vi "Decode Key.vi"(9 "PlatMods":T1, 10 "Mods":cluster{"Num Pad":bool, "Menu Key":bool}, 11 "ScanCode":i16) -> (3 "Key":string)   [LabVIEW 2021, in "Seq Edit Quick Drop.lvlib"]
uses:
  Seq Edit Quick Drop.lvlib
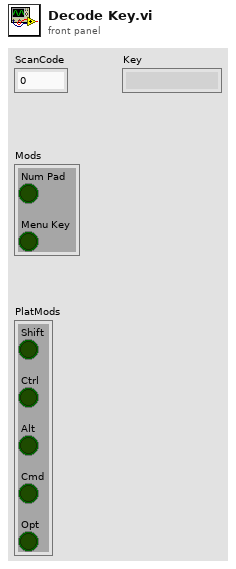
[diagram p1: front panel]
types:
  T1 = cluster{"Shift":bool, "Ctrl":bool, "Alt":bool, "Cmd":bool, "Opt":bool}
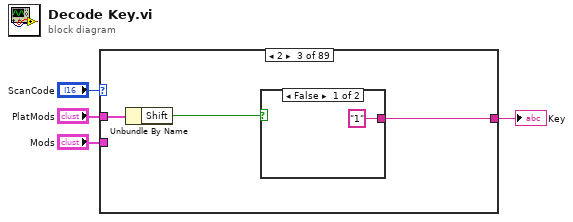
[diagram p0: block diagram]
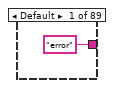
[diagram p2: hidden frame]
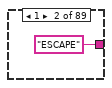
[diagram p3: hidden frame]
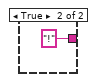
[diagram p4: hidden frame]
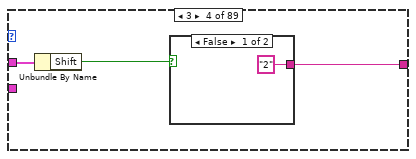
[diagram p5: hidden frame]
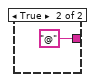
[diagram p6: hidden frame]
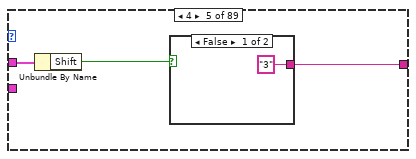
[diagram p7: hidden frame]
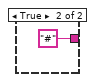
[diagram p8: hidden frame]
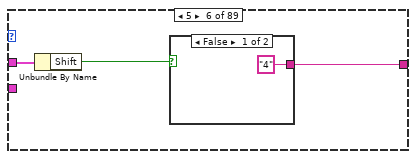
[diagram p9: hidden frame]
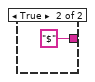
[diagram p10: hidden frame]
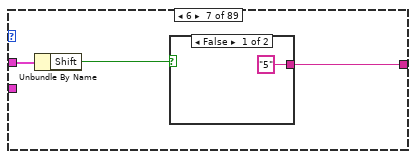
[diagram p11: hidden frame]
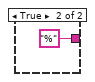
[diagram p12: hidden frame]
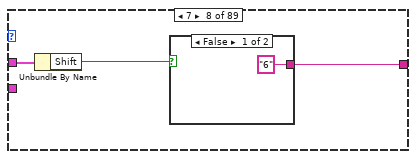
[diagram p13: hidden frame]
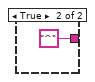
[diagram p14: hidden frame]
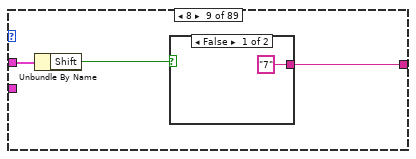
[diagram p15: hidden frame]
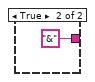
[diagram p16: hidden frame]
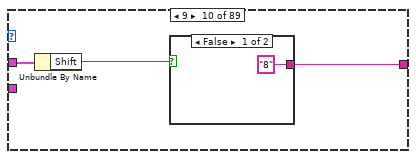
[diagram p17: hidden frame]
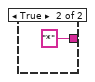
[diagram p18: hidden frame]
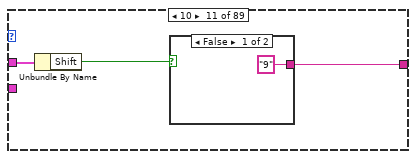
[diagram p19: hidden frame]
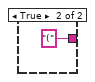
[diagram p20: hidden frame]
diagram:
  n1 = case shown="2" "ScanCode" {
    tunnel: ["error" "ESCAPE" w8 w13 w19 w24 w29 w32 w39 w44 w49 w54 w58 w62 "backspace" "tab" w70 w75 w80 w84 w89 w94 w99 w104 w109 w114 w119 w124 "Enter" "control" w132 w137 w142 w147 w152 w157 w162 w167 w172 w177 w181 w186 "LSHIFT" w193 w197 w203 w208 w212 w217 w222 w227 w232 w237 w243 "RSHIFT" w250 "RSHIFT" "SPACE" "CAPSLOCK" "F1" "F2" "F3" "F4" "F5" "F6" "F7" "F8" "F9" "F10" "numlock" "error" w269 w275 w278 "-" w284 "5" w290 "+" w296 w301 w306 w313 w318 "F11" "F12" "left win key" "right win key" "select"] -> w2
    tunnel: "Mods" -> [_ _ _ _ _ _ _ _ _ _ _ _ _ _ _ _ _ _ _ _ _ _ _ _ _ _ _ _ _ _ _ _ _ _ _ _ _ _ _ _ _ _ _ _ _ _ _ _ _ _ _ _ _ _ _ w248 _ _ _ _ _ _ _ _ _ _ _ _ _ _ _ w268 w274 w279 _ w285 _ w291 _ w297 w302 w307 w311 w316 _ _ _ _ _]
    tunnel: "PlatMods" -> [_ _ w9 w12 w17 w22 w27 w33 w37 w42 w47 w52 w57 w63 _ _ w69 w74 w79 w85 w90 w95 w100 w105 w110 w115 w120 w125 _ _ w131 w136 w141 w146 w151 w156 w161 w166 w171 w176 w182 w187 _ w192 w198 w202 w207 w213 w218 w223 w228 w233 w238 w242 _ _ _ _ _ _ _ _ _ _ _ _ _ _ _ _ _ _ _ _ _ _ _ _ _ _ _ _ _ _ _ _ _ _ _]
    frame Default {
    }
    frame 1 {
    }
    frame 2 {
      n2 = Unbundle By Name(w9) -> ("Shift"=w7:bool)
      n3 = case shown="False" w7 {
        tunnel: ["1" "!"] -> w8
        frame False {
        }
        frame True {
        }
      }
    }
    frame 3 {
      n4 = Unbundle By Name(w12) -> ("Shift"=w14:bool)
      n5 = case shown="False" w14 {
        tunnel: ["2" "@"] -> w13
        frame False {
        }
        frame True {
        }
      }
    }
    frame 4 {
      n6 = Unbundle By Name(w17) -> ("Shift"=w18:bool)
      n7 = case shown="False" w18 {
        tunnel: ["3" "#"] -> w19
        frame False {
        }
        frame True {
        }
      }
    }
    frame 5 {
      n8 = Unbundle By Name(w22) -> ("Shift"=w23:bool)
      n9 = case shown="False" w23 {
        tunnel: ["4" "$"] -> w24
        frame False {
        }
        frame True {
        }
      }
    }
    frame 6 {
      n10 = Unbundle By Name(w27) -> ("Shift"=w28:bool)
      n11 = case shown="False" w28 {
        tunnel: ["5" "%"] -> w29
        frame False {
        }
        frame True {
        }
      }
    }
    frame 7 {
      n12 = Unbundle By Name(w33) -> ("Shift"=w34:bool)
      n13 = case shown="False" w34 {
        tunnel: ["6" "^"] -> w32
        frame False {
        }
        frame True {
        }
      }
    }
    frame 8 {
      n14 = Unbundle By Name(w37) -> ("Shift"=w38:bool)
      n15 = case shown="False" w38 {
        tunnel: ["7" "&"] -> w39
        frame False {
        }
        frame True {
        }
      }
    }
    frame 9 {
      n16 = Unbundle By Name(w42) -> ("Shift"=w43:bool)
      n17 = case shown="False" w43 {
        tunnel: ["8" "*"] -> w44
        frame False {
        }
        frame True {
        }
      }
    }
    frame 10 {
      n18 = Unbundle By Name(w47) -> ("Shift"=w48:bool)
      n19 = case shown="False" w48 {
        tunnel: ["9" "("] -> w49
        frame False {
        }
        frame True {
        }
      }
    }
    frame 11 {
      n20 = Unbundle By Name(w52) -> ("Shift"=w53:bool)
      n21 = case shown="False" w53 {
        tunnel: ["0" ")"] -> w54
        frame False {
        }
        frame True {
        }
      }
    }
    frame 12 {
      n22 = Unbundle By Name(w57) -> ("Shift"=w59:bool)
      n23 = case shown="False" w59 {
        tunnel: ["-" "_"] -> w58
        frame False {
        }
        frame True {
        }
      }
    }
    frame 13 {
      n24 = Unbundle By Name(w63) -> ("Shift"=w64:bool)
      n25 = case shown="False" w64 {
        tunnel: ["=" "+"] -> w62
        frame False {
        }
        frame True {
        }
      }
    }
    frame 14 {
    }
    frame 15 {
    }
    frame 16 {
      n26 = Unbundle By Name(w69) -> ("Shift"=w71:bool)
      n27 = case shown="False" w71 {
        tunnel: ["q" "Q"] -> w70
        frame False {
        }
        frame True {
        }
      }
    }
    frame 17 {
      n28 = Unbundle By Name(w74) -> ("Shift"=w76:bool)
      n29 = case shown="False" w76 {
        tunnel: ["w" "W"] -> w75
        frame False {
        }
        frame True {
        }
      }
    }
    frame 18 {
      n30 = Unbundle By Name(w79) -> ("Shift"=w81:bool)
      n31 = case shown="False" w81 {
        tunnel: ["e" "E"] -> w80
        frame False {
        }
        frame True {
        }
      }
    }
    frame 19 {
      n32 = Unbundle By Name(w85) -> ("Shift"=w86:bool)
      n33 = case shown="False" w86 {
        tunnel: ["r" "R"] -> w84
        frame False {
        }
        frame True {
        }
      }
    }
    frame 20 {
      n34 = Unbundle By Name(w90) -> ("Shift"=w91:bool)
      n35 = case shown="False" w91 {
        tunnel: ["t" "T"] -> w89
        frame False {
        }
        frame True {
        }
      }
    }
    frame 21 {
      n36 = Unbundle By Name(w95) -> ("Shift"=w96:bool)
      n37 = case shown="False" w96 {
        tunnel: ["y" "Y"] -> w94
        frame False {
        }
        frame True {
        }
      }
    }
    frame 22 {
      n38 = Unbundle By Name(w100) -> ("Shift"=w101:bool)
      n39 = case shown="False" w101 {
        tunnel: ["u" "U"] -> w99
        frame False {
        }
        frame True {
        }
      }
    }
    frame 23 {
      n40 = Unbundle By Name(w105) -> ("Shift"=w106:bool)
      n41 = case shown="False" w106 {
        tunnel: ["i" "I"] -> w104
        frame False {
        }
        frame True {
        }
      }
    }
    frame 24 {
      n42 = Unbundle By Name(w110) -> ("Shift"=w111:bool)
      n43 = case shown="False" w111 {
        tunnel: ["o" "O"] -> w109
        frame False {
        }
        frame True {
        }
      }
    }
    frame 25 {
      n44 = Unbundle By Name(w115) -> ("Shift"=w116:bool)
      n45 = case shown="False" w116 {
        tunnel: ["p" "P"] -> w114
        frame False {
        }
        frame True {
        }
      }
    }
    frame 26 {
      n46 = Unbundle By Name(w120) -> ("Shift"=w121:bool)
      n47 = case shown="False" w121 {
        tunnel: ["[" "{"] -> w119
        frame False {
        }
        frame True {
        }
      }
    }
    frame 27 {
      n48 = Unbundle By Name(w125) -> ("Shift"=w126:bool)
      n49 = case shown="False" w126 {
        tunnel: ["}" "P"] -> w124
        frame False {
        }
        frame True {
        }
      }
    }
    frame 28 {
    }
    frame 29 {
    }
    frame 30 {
      n50 = Unbundle By Name(w131) -> ("Shift"=w133:bool)
      n51 = case shown="False" w133 {
        tunnel: ["a" "A"] -> w132
        frame False {
        }
        frame True {
        }
      }
    }
    frame 31 {
      n52 = Unbundle By Name(w136) -> ("Shift"=w138:bool)
      n53 = case shown="False" w138 {
        tunnel: ["s" "S"] -> w137
        frame False {
        }
        frame True {
        }
      }
    }
    frame 32 {
      n54 = Unbundle By Name(w141) -> ("Shift"=w143:bool)
      n55 = case shown="False" w143 {
        tunnel: ["d" "D"] -> w142
        frame False {
        }
        frame True {
        }
      }
    }
    frame 33 {
      n56 = Unbundle By Name(w146) -> ("Shift"=w148:bool)
      n57 = case shown="False" w148 {
        tunnel: ["f" "F"] -> w147
        frame False {
        }
        frame True {
        }
      }
    }
    frame 34 {
      n58 = Unbundle By Name(w151) -> ("Shift"=w153:bool)
      n59 = case shown="False" w153 {
        tunnel: ["g" "G"] -> w152
        frame False {
        }
        frame True {
        }
      }
    }
    frame 35 {
      n60 = Unbundle By Name(w156) -> ("Shift"=w158:bool)
      n61 = case shown="False" w158 {
        tunnel: ["h" "H"] -> w157
        frame False {
        }
        frame True {
        }
      }
    }
    frame 36 {
      n62 = Unbundle By Name(w161) -> ("Shift"=w163:bool)
      n63 = case shown="False" w163 {
        tunnel: ["j" "J"] -> w162
        frame False {
        }
        frame True {
        }
      }
    }
    frame 37 {
      n64 = Unbundle By Name(w166) -> ("Shift"=w168:bool)
      n65 = case shown="False" w168 {
        tunnel: ["k" "K"] -> w167
        frame False {
        }
        frame True {
        }
      }
    }
    frame 38 {
      n66 = Unbundle By Name(w171) -> ("Shift"=w173:bool)
      n67 = case shown="False" w173 {
        tunnel: ["l" "L"] -> w172
        frame False {
        }
        frame True {
        }
      }
    }
    frame 39 {
      n68 = Unbundle By Name(w176) -> ("Shift"=w178:bool)
      n69 = case shown="False" w178 {
        tunnel: [";" ":"] -> w177
        frame False {
        }
        frame True {
        }
      }
    }
    frame 40 {
      n70 = Unbundle By Name(w182) -> ("Shift"=w183:bool)
      n71 = case shown="False" w183 {
        tunnel: ["'" "\""] -> w181
        frame False {
        }
        frame True {
        }
      }
    }
    frame 41 {
      n72 = Unbundle By Name(w187) -> ("Shift"=w188:bool)
      n73 = case shown="False" w188 {
        tunnel: ["`" "~"] -> w186
        frame False {
        }
        frame True {
        }
      }
    }
    frame 42 {
    }
    frame 43 {
      n74 = Unbundle By Name(w192) -> ("Shift"=w194:bool)
      n75 = case shown="False" w194 {
        tunnel: [";" ":"] -> w193
        frame False {
        }
        frame True {
        }
      }
    }
    frame 44 {
      n76 = Unbundle By Name(w198) -> ("Shift"=w199:bool)
      n77 = case shown="False" w199 {
        tunnel: ["z" "Z"] -> w197
        frame False {
        }
        frame True {
        }
      }
    }
    frame 45 {
      n78 = Unbundle By Name(w202) -> ("Shift"=w204:bool)
      n79 = case shown="False" w204 {
        tunnel: ["x" "X"] -> w203
        frame False {
        }
        frame True {
        }
      }
    }
    frame 46 {
      n80 = Unbundle By Name(w207) -> ("Shift"=w209:bool)
      n81 = case shown="False" w209 {
        tunnel: ["c" "C"] -> w208
        frame False {
        }
        frame True {
        }
      }
    }
    frame 47 {
      n82 = Unbundle By Name(w213) -> ("Shift"=w214:bool)
      n83 = case shown="False" w214 {
        tunnel: ["v" "V"] -> w212
        frame False {
        }
        frame True {
        }
      }
    }
    frame 48 {
      n84 = Unbundle By Name(w218) -> ("Shift"=w219:bool)
      n85 = case shown="False" w219 {
        tunnel: ["b" "B"] -> w217
        frame False {
        }
        frame True {
        }
      }
    }
    frame 49 {
      n86 = Unbundle By Name(w223) -> ("Shift"=w224:bool)
      n87 = case shown="False" w224 {
        tunnel: ["n" "N"] -> w222
        frame False {
        }
        frame True {
        }
      }
    }
    frame 50 {
      n88 = Unbundle By Name(w228) -> ("Shift"=w229:bool)
      n89 = case shown="False" w229 {
        tunnel: ["m" "M"] -> w227
        frame False {
        }
        frame True {
        }
      }
    }
    frame 51 {
      n90 = Unbundle By Name(w233) -> ("Shift"=w234:bool)
      n91 = case shown="False" w234 {
        tunnel: ["," "<"] -> w232
        frame False {
        }
        frame True {
        }
      }
    }
    frame 52 {
      n92 = Unbundle By Name(w238) -> ("Shift"=w239:bool)
      n93 = case shown="False" w239 {
        tunnel: ["." ">"] -> w237
        frame False {
        }
        frame True {
        }
      }
    }
    frame 53 {
      n94 = Unbundle By Name(w242) -> ("Shift"=w244:bool)
      n95 = case shown="False" w244 {
        tunnel: ["/" "?"] -> w243
        frame False {
        }
        frame True {
        }
      }
    }
    frame 54 {
    }
    frame 55 {
      n96 = Unbundle By Name(w248) -> ("Num Pad"=w249:bool)
      n97 = case shown="False" w249 {
        tunnel: ["PRINTSCREEN" "/"] -> w250
        frame False {
        }
        frame True {
        }
      }
    }
    frame 56 {
    }
    frame 57 {
    }
    frame 58 {
    }
    frame 59 {
    }
    frame 60 {
    }
    frame 61 {
    }
    frame 62 {
    }
    frame 63 {
    }
    frame 64 {
    }
    frame 65 {
    }
    frame 66 {
    }
    frame 67 {
    }
    frame 68 {
    }
    frame 69 {
    }
    frame 70 {
    }
    frame 71 {
      n98 = Unbundle By Name(w268) -> ("Num Pad"=w270:bool)
      n99 = case shown="False" w270 {
        tunnel: ["HOME" "7"] -> w269
        frame False {
        }
        frame True {
        }
      }
    }
    frame 72 {
      n100 = Unbundle By Name(w274) -> ("Num Pad"=w273:bool)
      n101 = case shown="False" w273 {
        tunnel: ["UP" "8"] -> w275
        frame False {
        }
        frame True {
        }
      }
    }
    frame 73 {
      n102 = Unbundle By Name(w279) -> ("Num Pad"=w280:bool)
      n103 = case shown="False" w280 {
        tunnel: ["PAGEUP" "9"] -> w278
        frame False {
        }
        frame True {
        }
      }
    }
    frame 74 {
    }
    frame 75 {
      n104 = Unbundle By Name(w285) -> ("Num Pad"=w286:bool)
      n105 = case shown="False" w286 {
        tunnel: ["LEFT" "4"] -> w284
        frame False {
        }
        frame True {
        }
      }
    }
    frame 76 {
    }
    frame 77 {
      n106 = Unbundle By Name(w291) -> ("Num Pad"=w292:bool)
      n107 = case shown="False" w292 {
        tunnel: ["RIGHT" "6"] -> w290
        frame False {
        }
        frame True {
        }
      }
    }
    frame 78 {
    }
    frame 79 {
      n108 = Unbundle By Name(w297) -> ("Num Pad"=w298:bool)
      n109 = case shown="False" w298 {
        tunnel: ["END" "1"] -> w296
        frame False {
        }
        frame True {
        }
      }
    }
    frame 80 {
      n110 = Unbundle By Name(w302) -> ("Num Pad"=w303:bool)
      n111 = case shown="False" w303 {
        tunnel: ["DOWN" "2"] -> w301
        frame False {
        }
        frame True {
        }
      }
    }
    frame 81 {
      n112 = Unbundle By Name(w307) -> ("Num Pad"=w308:bool)
      n113 = case shown="False" w308 {
        tunnel: ["PAGEDOWN" "3"] -> w306
        frame False {
        }
        frame True {
        }
      }
    }
    frame 82 {
      n114 = Unbundle By Name(w311) -> ("Num Pad"=w312:bool)
      n115 = case shown="False" w312 {
        tunnel: ["INSERT" "0"] -> w313
        frame False {
        }
        frame True {
        }
      }
    }
    frame 83 {
      n116 = Unbundle By Name(w316) -> ("Num Pad"=w317:bool)
      n117 = case shown="False" w317 {
        tunnel: ["DELETE" "."] -> w318
        frame False {
        }
        frame True {
        }
      }
    }
    frame 87 {
    }
    frame 88 {
    }
    frame 91 {
    }
    frame 92 {
    }
    frame 93 {
    }
  }
  "Key" <- w2
